vi "RampRateCoordinated.vi"(6 "return immediately":bool, 7 "ramp rate":dbl, 8 "error in (no error)":T1, 9 "taskId":i32(ring) items=["TLibrary", "T01", "T02", "T03", "T04", "T05", "T06", "T07", "T08", "T09", "T10", "T11", "T12", "T13", "T14", "T15", "T16", "T17", "T18", "T19", "T20", "T21", "T22", "T23", "T24", "T25", "T26", "T27", "T28", "T29", "T30", "T31"], 11 "controller in":refnum<k24>) -> (0 "error out":T1, 3 "controller out":refnum<k24>)   [LabVIEW 2020, in "Aerotech.lvlib"]
doc: "Acceleration and Deceleration rates are set to ramp rate for coordinated moves."
uses:
  Aerotech.lvlib
  C:/Users/HEP/Documents/GitHub/UCSB-Gantry-HEP/Drivers/Aerotech A3200/Bin/Aerotech.A3200.LabVIEW.dll
  UCSB-Gantry-HEP/Drivers/Aerotech A3200/Bin/Aerotech.A3200.LabVIEW.dll
  C:/Program Files (x86)/Aerotech/A3200/LabVIEW/2010/Bin/Aerotech.A3200.dll
  Program Files (x86)/Aerotech/A3200/LabVIEW/2010/Bin/Aerotech.A3200.dll
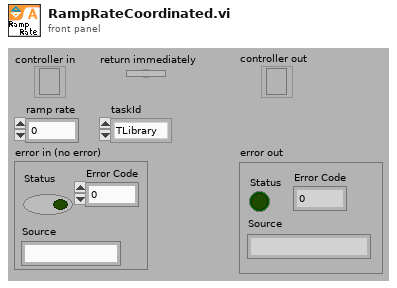
[diagram p1: front panel]
types:
  T1 = cluster{"Status":bool, "Error Code":i32, "Source":string}
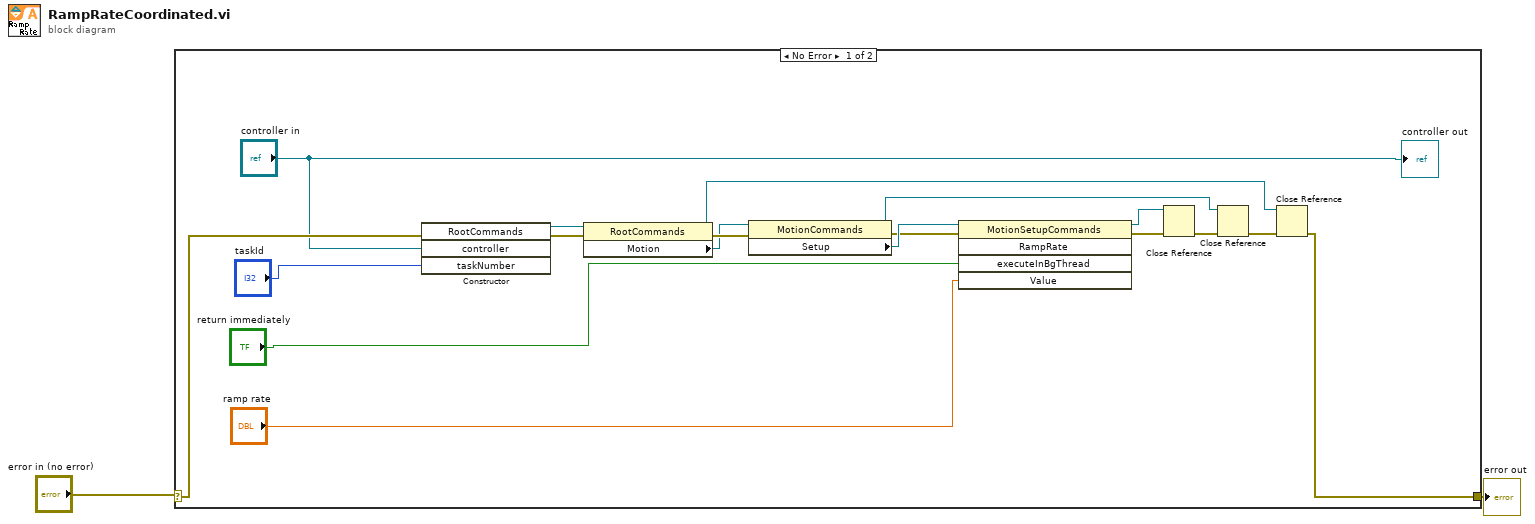
[diagram p0: block diagram]
diagram:
  n1 = case shown="No Error" "error in (no error)" {
    selector: "error in (no error)" -> [w20 w21]
    tunnel: [w4 w21] -> w1
    frame No Error {
      n2 = constructor class="RootCommands"(error in=w20, "controller"="controller in", "taskNumber"="taskId") -> (reference out=w17:refnum<k24>, error out=w18:errorcluster)  [unwired: 2 in, 3 out]
      n3 = property class="RootCommands"(reference=w17, error in=w18) -> (reference out=w5:refnum<k24>, error out=w16:errorcluster, "Motion"=w15:refnum<k24>)
      n4 = property class="MotionCommands"(reference=w15, error in=w16) -> (reference out=w7:refnum<k24>, error out=w13:errorcluster, "Setup"=w14:refnum<k24>)
      n5 = invoke class="MotionSetupCommands" method="RampRate"(reference=w14, error in=w13, "executeInBgThread"="return immediately", "Value"="ramp rate") -> (reference out=w9:refnum<k24>, error out=w10:errorcluster)  [unwired: 1 in, 3 out]
      n6 = Close Reference(reference=w9, error in (no error)=w10) -> (error out=w8:errorcluster)
      n7 = Close Reference(reference=w7, error in (no error)=w8) -> (error out=w6:errorcluster)
      n8 = Close Reference(reference=w5, error in (no error)=w6) -> (error out=w4:errorcluster)
      "controller out" <- "controller in"
    }
    frame Error {
    }
  }
  "error out" <- w1
